vi "Finite Analog Sampling Example.vi"() -> ()   [LabVIEW 2015, in "LabVIEW Interface for Arduino.lvlib"]
doc: "This example acquires a finite number of samples from an Analog Input."
uses:
  <vilib>/LabVIEW Interface for Arduino/LabVIEW Interface for Arduino.lvlib
panel:
  in  "Analog Input Pin":u8
  out "Data":waveform(dbl)(graph)
  in  "Acquition Speed (HZ)":u16=500
  in  "Number of Samples":u16
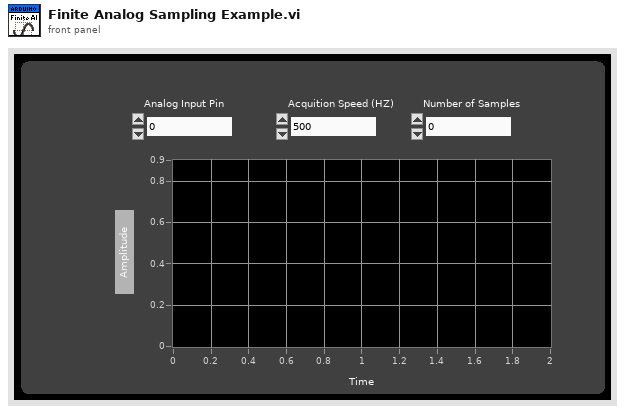
[diagram p1: front panel]
types:
  T1 = typedef "LabVIEW Interface for Arduino.lvlib/Arduino Resource.ctl" = cluster{"VISA resource":refnum<visa-resource-name>, "Board Type":T2, "Connection Type":enum8{"USB / Serial"}, "Bytes Per Packet (15)":u8}
  T2 = typedef "LabVIEW Interface for Arduino.lvlib/Board Type.ctl" = enum16{"Uno", "Dimuelanove w/Atmega 328", "Mega 2560"}
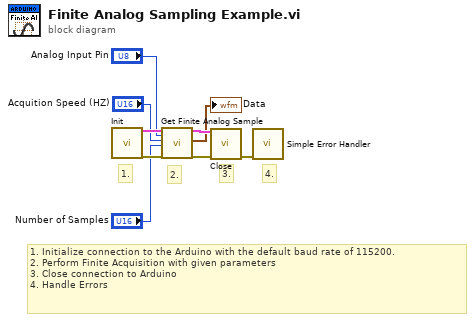
[diagram p0: block diagram]
diagram:
  # "4."
  # "3."
  # "2."
  # "1."
  # "1. Initialize connection to the Arduino with the default baud rate of 115200.\n2. Perform Finite Acquisition with given parameters\n3. Close connection to Arduino\n4. Handle Errors"
  n1 = call <vilib>:"Init.vi"() -> ("Arduino Resource"=w9:T1, "error out"=w5:errorcluster)  [unwired: 18 in]
  n2 = call <vilib>:"Get Finite Analog Sample.vi"("Arduino Resource"=w9, "Analog Input Pin"="Analog Input Pin", "Acquition Speed (HZ)"="Acquition Speed (HZ)", "Number of Samples"="Number of Samples", "error in"=w5) -> ("Arduino Resource"=w8:T1, "Data"=→"Data":waveform(dbl), "error out"=w6:errorcluster)  [unwired: 11 in, 1 out]
  n3 = call <vilib>:"Close.vi"("Arduino Resource"=w8, "error in"=w6) -> ("error out"=w7:errorcluster)  [unwired: 13 in]
  n4 = call <vilib>:"Simple Error Handler.vi"("error in (no error)"=w7) -> ()  [unwired: 4 in, 5 out]
